vi "URAPI_ReadAnalogIn.vi"(0 "Variable In":string="voltage", 3 "URAPI Script":T1={"Script"="", "Whiles"=[], "Ifs"=[], "Supress Err"=TRUE, "Errors"=""}, 4 "Channel":string) -> (2 "Variable Out":string, 5 "URAPI Script":T1={"Script"="", "Whiles"=[], "Ifs"=[], "Supress Err"=TRUE, "Errors"=""})   [LabVIEW 2012]
doc: "Reads the value of the specified analog \"Channel\" and returns that value as \"Variable Out\"."
uses:
  <userlib>/BotSpeak/VIs/Direct/URAPI_Control.ctl
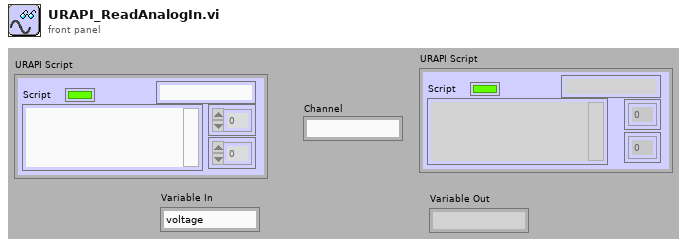
[diagram p1: front panel]
types:
  T1 = typedef "URAPI_Control.ctl" = cluster{"Script":string, "Whiles":u8[], "Ifs":u8[], "Supress Err":bool, "Errors":string}
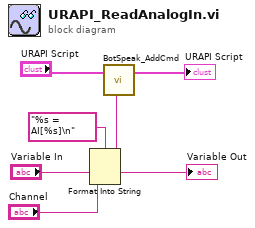
[diagram p0: block diagram]
diagram:
  n1 = Format Into String(format string="%s = AI[%s]\n" ("string"), "Variable In", "Channel") -> (resulting string=w2:string)  [unwired: 2 in, 1 out]
  n2 = call <userlib>:"BotSpeak_AddCmd.vi"("String"=w2, "URAPI Script"="URAPI Script") -> ("URAPI Script out"=→"URAPI Script":T1)  [unwired: 1 in]
  "Variable Out" <- "Variable In"
